vi "MISC Wait on Abort Notifier.vi"(7 "Notifier":refnum<notifier>, 8 "Error In (no error)":errorcluster, 11 "Wait Time (500ms)":u32=500) -> (0 "Error Out":errorcluster, 1 "Aborted":bool, 2 "Notification":string, 3 "Timer Value (ms)":u32)   [LabVIEW 2011]
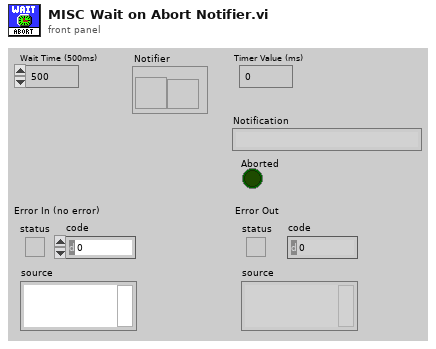
[diagram p1: front panel]
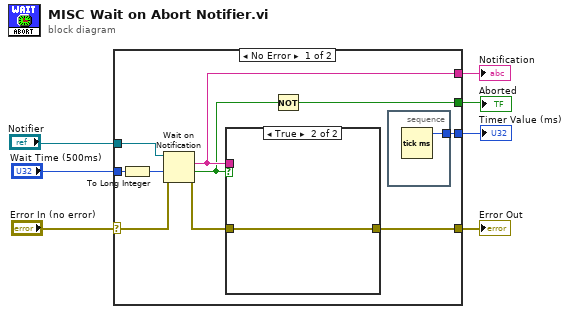
[diagram p0: block diagram]
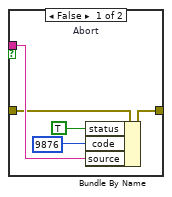
[diagram p2: hidden frame]
diagram:
  n1 = case shown="No Error" "Error In (no error)" {
    selector: "Error In (no error)" -> [w12 w25]
    tunnel: "Wait Time (500ms)" -> [w14 _]
    tunnel: [w11 w25] -> w6
    tunnel: "Notifier" -> [w17 _]
    tunnel: [w8 _] -> w5
    tunnel: [w16 _] -> w4
    tunnel: [w10 _] -> w1
    frame No Error {
      n2 = To Long Integer(number=w14) -> (32bit integer=w15:i32)
      n3 = Wait on Notification(notifier=w17, timeout in ms (-1)=w15, error in (no error)=w12) -> (notification=w10:string, timed out?=w9:bool, error out=w13:errorcluster)  [unwired: 2 out]
      n4 = case shown="True" w9 {
        tunnel: w13 -> [w19 w23]
        tunnel: [w18 w23] -> w11
        tunnel: w10 -> [w22 _]
        frame False {
          w20 = 9876  # Abort
          n5 = Bundle By Name(cluster=w19, "status"=TRUE, "code"=w20, "source"=w22) -> (w18:errorcluster)
        }
        frame True {
        }
      }
      n6 = Not(x=w9) -> (.not. x?=w8:bool)
      n7 = stacked-sequence {
        tunnel: [w24] -> w16
        frame #0 {
          n8 = Tick Count (ms)() -> (millisecond timer value=w24:u32)
        }
      }
    }
    frame Error {
    }
  }
  "Error Out" <- w6
  "Aborted" <- w5
  "Timer Value (ms)" <- w4
  "Notification" <- w1
